vi "medAFMprel.vi"(6 "stop":bool, 8 "error in (no error)":errorcluster, 9 "Tipo":enum16{"Amplitud", "Fase", "Mixto"}(ring), 10 "thrAng":dbl=4.0 format="%#_13g", 11 "thr":dbl) -> (0 "error out":errorcluster, 2 "posicion":dbl)   [LabVIEW 2018]
uses:
  <vilib>/Analysis/NI_AALPro.lvlib
panel:
  out "Cerca":bool
  in  "NUMERO DE MED.":i32=1 min=1 max=10
  in  "wait afm":u32=300
  out "Amplitud":dbl[](graph)=[0.0001737, 0.0001907, 0.0001951, 0.0001957, 0.0001958, 0.0001961, 0.0001961, 0.000196, 0.0001957, 0.0001957, 0.000196, 0.000196, 0.0001958, 0.000196, 0.000196, 0.0001958, 0.0001957, 0.0001957, 0.000196, 0.0001963, 0.0001963, 0.0001966, 0.0001966, 0.0001963, 0.0001965, 0.0001967, 0.0001966, 0.0001966, 0.0001966, 0.0001968, 0.000197, 0.000197, 0.000197, 0.0001968, 0.0001967, 0.0001967, 0.0001966, 0.0001966, 0.0001962, 0.000196, 0.0001961, 0.0001963, 0.0001962, 0.0001962, 0.0001962, 0.0001963, 0.0001965, 0.0001963, 0.0001962, 0.0001961, 0.0001958, 0.0001958, 0.0001958, 0.0001957, 0.0001955, 0.0001955, 0.000196, 0.0001961, 0.0001958, 0.0001956, 0.000196, 0.0001958, 0.0001958, 0.000196, 0.0001958, 0.000196, 0.0001958, 0.0001958, 0.0001958, 0.0001956, 0.0001952, 0.0001952, 0.0001956, 0.0001956, 0.0001957, 0.0001956, 0.0001955, 0.0001958, 0.0001958, 0.0001961, 0.0001962, 0.0001962, 0.0001963, 0.0001966, 0.0001965, 0.0001966, 0.0001966, 0.0001968, 0.0001968, 0.0001966, 0.0001961, 0.0001962, 0.0001965, 0.0001967, 0.0001963, 0.0001961, 0.0001958, 0.0001963, 0.0001966, 0.0001965, 0.0001963, 0.0001961, 0.0001961, 0.0001966, 0.0001968, 0.0001967, 0.0001963, 0.0001961, 0.0001961, 0.0001961, 0.0001958, 0.0001957, 0.0001956, 0.0001957, 0.0001955, 0.0001956, 0.0001958, 0.0001952, 0.0001958, 0.0001958, 0.0001955, 0.0001955, 0.0001955, 0.0001961, 0.0001963, 0.0001965, 0.0001962, 0.000196, 0.0001963, 0.0001966, 0.0001966, 0.0001966, 0.0001963, 0.0001963, 0.0001966, 0.0001966, 0.0001966, 0.0001965, 0.0001963, 0.0001966, 0.0001967, 0.0001968, 0.0001967, 0.0001966, 0.0001966, 0.0001967, 0.0001966, 0.0001965, 0.0001963, 0.0001967, 0.0001963, 0.0001961, 0.0001956, 0.0001956, 0.0001956, 0.0001956, 0.0001955, 0.0001952, 0.0001952, 0.0001952, 0.0001955, 0.0001957, 0.0001956, 0.0001956, 0.0001956, 0.0001957, 0.0001958, 0.0001958, 0.0001956, 0.0001955, 0.0001956, 0.0001958, 0.0001957, 0.0001956, 0.0001956, 0.0001956, 0.0001958, 0.0001957, 0.0001955, 0.0001956, 0.000196, 0.0001958, 0.0001961, 0.000196, 0.000196, 0.0001958, 0.0001965, 0.0001963, 0.0001966, 0.0001965, 0.0001965, 0.0001965, 0.0001963, 0.0001963, 0.0001961, 0.0001961, 0.0001966, 0.0001966, 0.0001966, 0.0001965, 0.0001958, 0.000196, 0.0001962, 0.0001962, 0.0001965, 0.0001962, 0.0001963, 0.0001965, 0.0001963, 0.0001965, 0.0001961, 0.0001961, 0.0001961, 0.0001961, 0.0001962, 0.000196, 0.0001956, 0.0001961, 0.0001961, 0.0001958, 0.0001956, 0.0001953, 0.0001953, 0.0001956, 0.0001956, 0.0001953, 0.0001953, 0.0001955, 0.0001956, 0.0001955, 0.0001953, 0.0001952, 0.0001952, 0.0001957, 0.0001958, 0.0001958, 0.0001958, 0.0001958, 0.0001958, 0.0001958, 0.0001956, 0.0001955, 0.0001957, 0.000196, 0.0001961, 0.0001958, 0.0001957, 0.0001957, 0.0001958, 0.0001961, 0.0001961, 0.0001961, 0.0001958, 0.0001958, 0.0001961, 0.0001965, 0.0001963, 0.0001965, 0.0001965, 0.0001965, 0.0001962, 0.0001963, 0.0001963, 0.0001961, 0.0001961, 0.0001958, 0.0001958, 0.000196, 0.0001958, 0.0001955, 0.0001956, 0.0001958, 0.0001956, 0.0001955, 0.0001957, 0.0001958, 0.0001958, 0.0001958, 0.0001956, 0.0001953, 0.0001953, 0.0001955, 0.0001953, 0.000195, 0.0001947, 0.0001948, 0.0001951, 0.0001951, 0.000195, 0.0001946, 0.0001948, 0.0001948, 0.0001952, 0.000195, 0.000195, 0.0001953, 0.0001956, 0.0001956, 0.0001958, 0.0001958, 0.0001961, 0.0001961, 0.000196, 0.0001958, 0.000196, 0.0001962, 0.0001965, 0.0001961, 0.000196, 0.0001955, 0.0001975, 0.0001981, 0.0001973, 0.0001966, 0.0001957, 0.0001953, 0.0001948, 0.0001946, 0.0001942, 0.0001933, 0.0001905, 0.0001845, 0.0001812, 0.0001717]
  out "Fase":dbl[](graph)=[1.35, -1.7, -2.3, -2.4, -2.4, -2.4, -2.35, -2.4, -2.4, -2.45, -2.45, -2.45, -2.45, -2.4, -2.4, -2.4, -2.4, -2.4, -2.45, -2.4, -2.4, -2.4, -2.4, -2.4, -2.45, -2.45, -2.45, -2.45, -2.5, -2.45, -2.4, -2.45, -2.4, -2.4, -2.4, -2.4, -2.45, -2.4, -2.45, -2.5, -2.5, -2.5, -2.45, -2.45, -2.5, -2.5, -2.45, -2.45, -2.45, -2.45, -2.45, -2.45, -2.45, -2.45, -2.5, -2.5, -2.45, -2.45, -2.45, -2.5, -2.5, -2.45, -2.4, -2.4, -2.4, -2.4, -2.45, -2.45, -2.45, -2.45, -2.5, -2.45, -2.45, -2.45, -2.4, -2.45, -2.5, -2.45, -2.5, -2.5, -2.55, -2.45, -2.45, -2.45, -2.45, -2.45, -2.45, -2.45, -2.45, -2.4, -2.45, -2.45, -2.45, -2.45, -2.45, -2.55, -2.6, -2.5, -2.5, -2.45, -2.5, -2.55, -2.6, -2.55, -2.45, -2.45, -2.45, -2.5, -2.5, -2.55, -2.45, -2.45, -2.45, -2.55, -2.5, -2.45, -2.55, -2.55, -2.5, -2.45, -2.5, -2.5, -2.5, -2.5, -2.45, -2.45, -2.45, -2.55, -2.55, -2.5, -2.5, -2.5, -2.55, -2.55, -2.5, -2.5, -2.5, -2.55, -2.55, -2.55, -2.55, -2.55, -2.55, -2.45, -2.55, -2.5, -2.5, -2.45, -2.5, -2.55, -2.5, -2.5, -2.55, -2.55, -2.55, -2.55, -2.55, -2.6, -2.65, -2.6, -2.55, -2.45, -2.45, -2.5, -2.55, -2.55, -2.55, -2.55, -2.5, -2.6, -2.55, -2.65, -2.55, -2.55, -2.55, -2.5, -2.6, -2.55, -2.55, -2.6, -2.6, -2.6, -2.55, -2.6, -2.6, -2.6, -2.65, -2.6, -2.55, -2.55, -2.55, -2.55, -2.5, -2.55, -2.6, -2.65, -2.7, -2.65, -2.65, -2.65, -2.7, -2.7, -2.6, -2.65, -2.65, -2.65, -2.6, -2.6, -2.55, -2.65, -2.65, -2.6, -2.6, -2.55, -2.55, -2.55, -2.6, -2.6, -2.55, -2.6, -2.6, -2.65, -2.6, -2.65, -2.55, -2.6, -2.55, -2.55, -2.6, -2.6, -2.6, -2.65, -2.6, -2.6, -2.6, -2.6, -2.65, -2.6, -2.6, -2.5, -2.55, -2.6, -2.7, -2.65, -2.6, -2.65, -2.7, -2.7, -2.7, -2.6, -2.55, -2.55, -2.6, -2.65, -2.6, -2.55, -2.6, -2.7, -2.7, -2.65, -2.6, -2.6, -2.6, -2.6, -2.55, -2.6, -2.65, -2.6, -2.65, -2.55, -2.5, -2.5, -2.55, -2.55, -2.6, -2.6, -2.65, -2.65, -2.6, -2.65, -2.65, -2.65, -2.65, -2.7, -2.65, -2.6, -2.6, -2.55, -2.55, -2.55, -2.65, -2.6, -2.65, -2.6, -2.65, -2.65, -2.65, -2.65, -2.65, -2.65, -2.6, -2.6, -2.6, -2.65, -2.65, -2.7, -2.65, -2.6, -2.55, 1.85, 14.25, 17.75, 19.65, 21.45, 22.75, 23.6, 24.45, 25.2, 25.05, 23.35, 15.35, 3.05, 0.4, 7.4]
  out "err R":dbl=0.1226366888094022
  out "diff Ph":dbl=9.8
  out "Z":dbl
  in  "controlP":T1
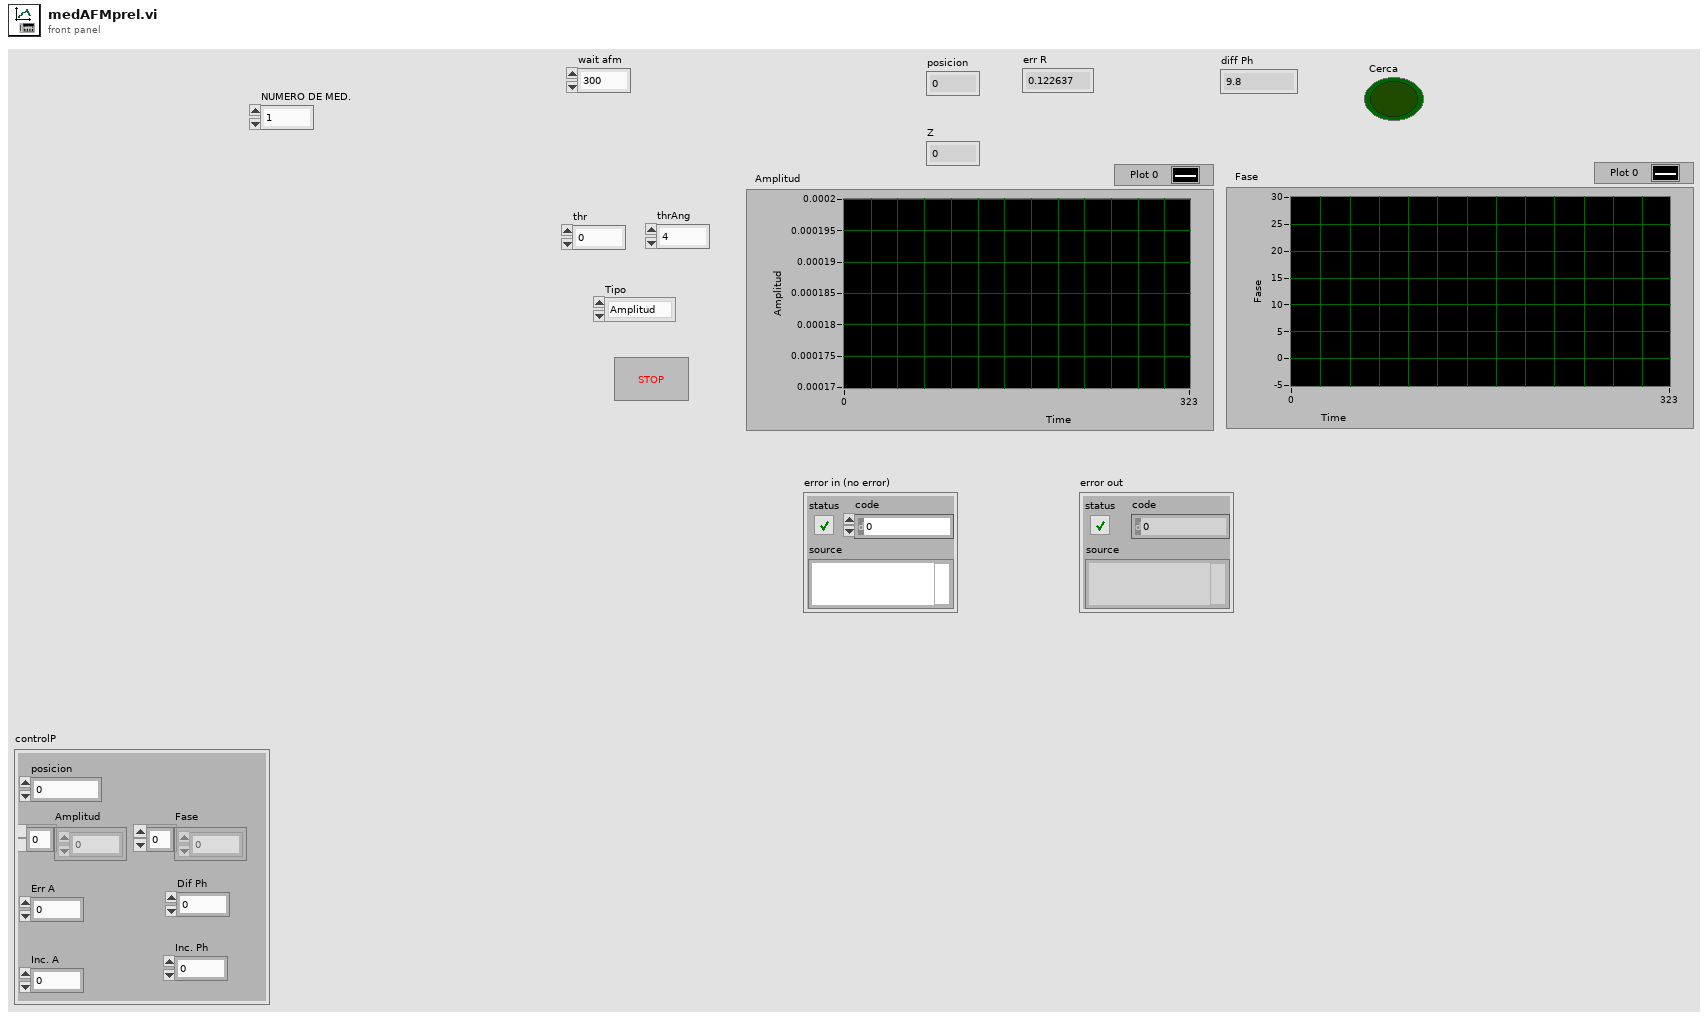
[diagram p1: front panel]
types:
  T1 = cluster{"posicion":dbl, "Amplitud":dbl[], "Fase":dbl[], "Err A":dbl, "Dif Ph":dbl, "Inc. A":dbl, "Inc. Ph":dbl}
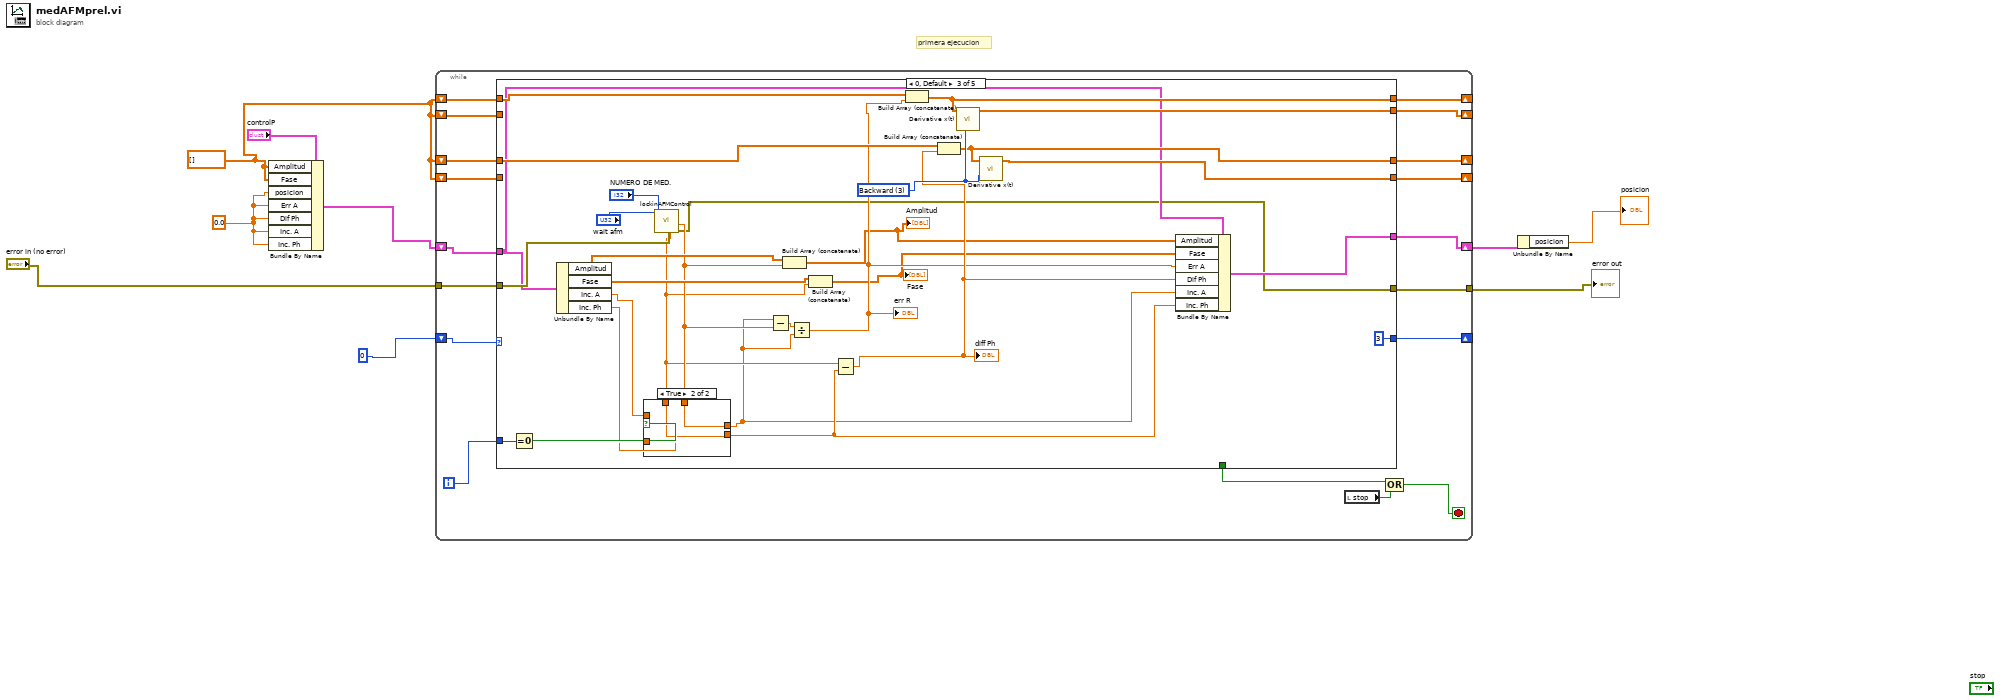
[diagram p0: block diagram]
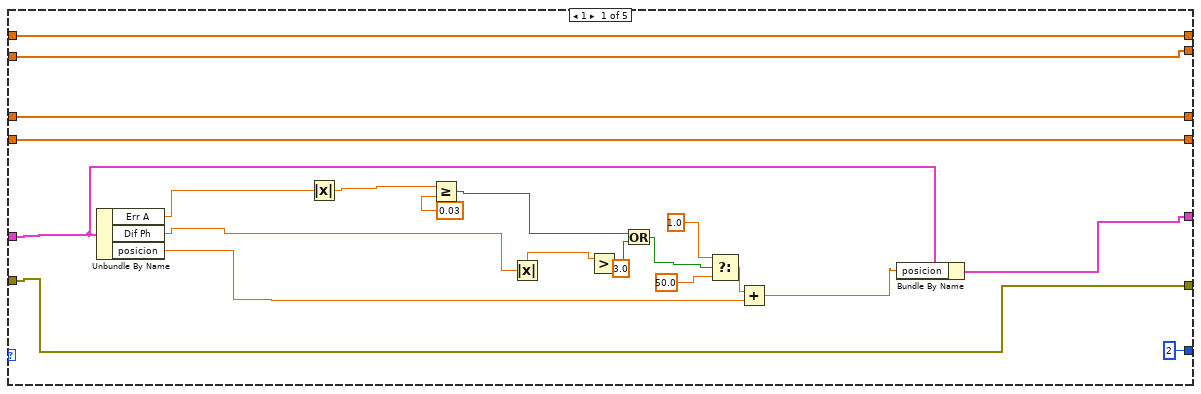
[diagram p2: hidden frame]
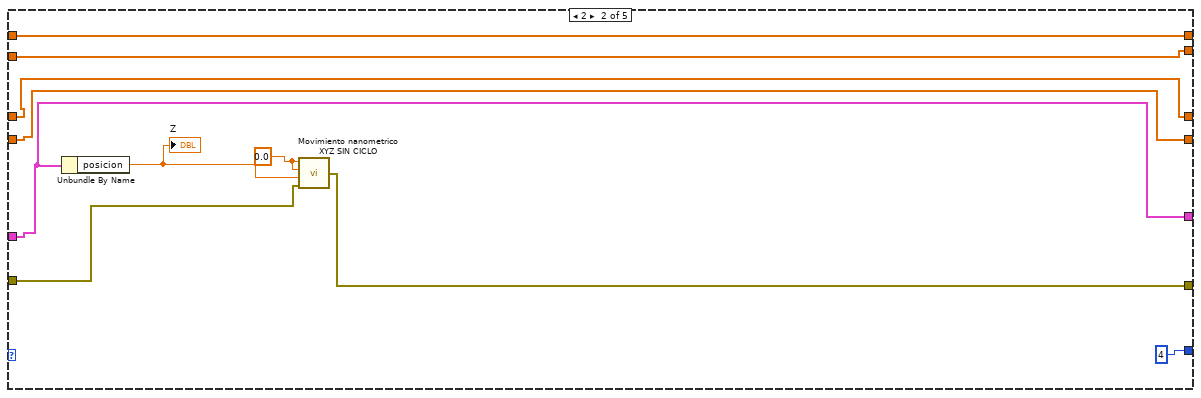
[diagram p3: hidden frame]
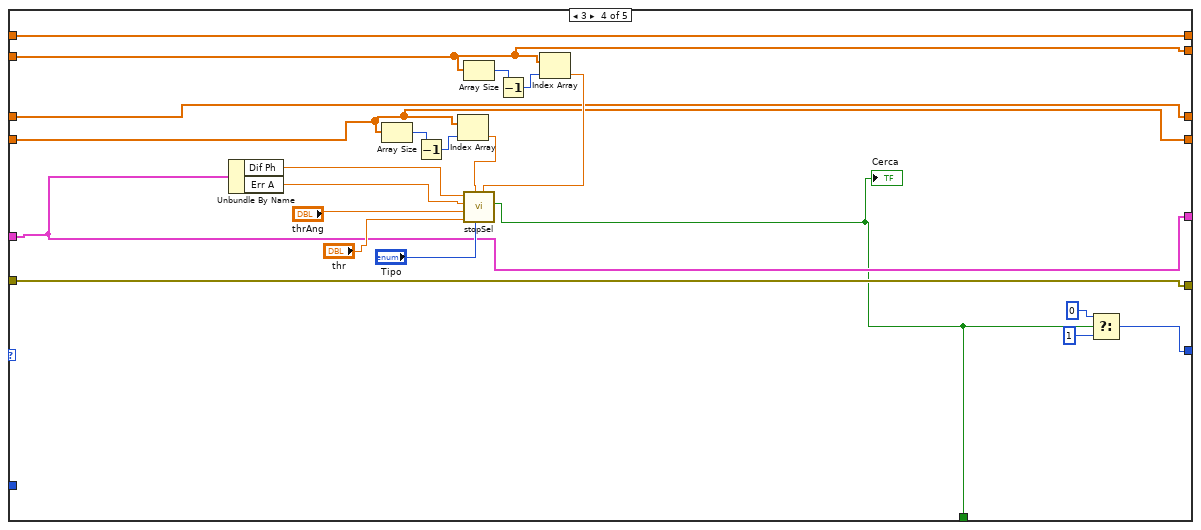
[diagram p5: hidden frame]
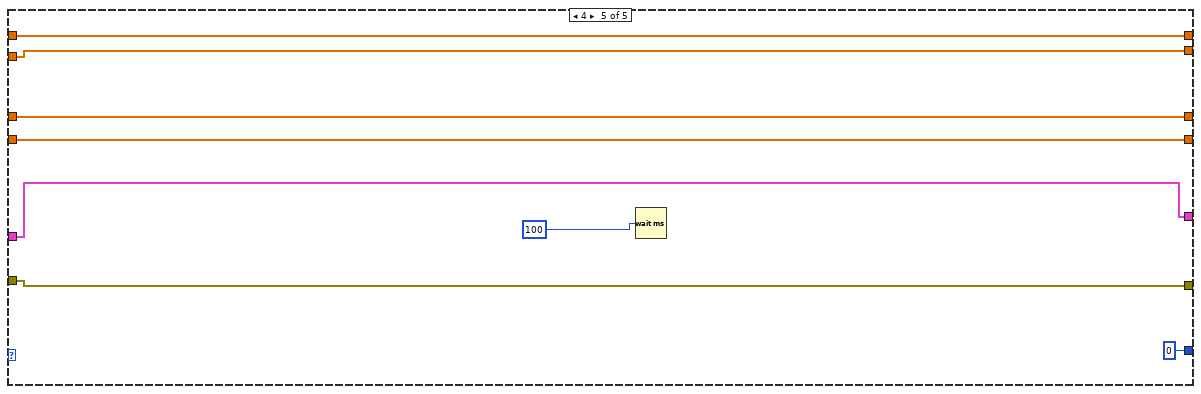
[diagram p6: hidden frame]
diagram:
  w6 = dbl[] []
  w8 = 0.0
  # "primera ejecucion"
  n1 = Bundle By Name(cluster="controlP", "Amplitud"=w6, "Fase"=w6, "posicion"=w8, "Err A"=w8, "Dif Ph"=w8, "Inc. A"=w8, "Inc. Ph"=w8) -> (w7:T1)
  n2 = while {
    shift-right: [w21] -> w4
    shift-left: w7 -> [w26]
    shift-right: [w16] -> _
    shift-left: w6 -> [w22]
    shift-right: [w15] -> _
    shift-left: w6 -> [w23]
    shift-right: [w14] -> _
    shift-left: w6 -> [w24]
    shift-right: [w13] -> _
    shift-left: w6 -> [w25]
    shift-right: [w18] -> _
    shift-left: 0 -> [w27]
    tunnel: "error in (no error)" -> [w20]
    tunnel: [w19] -> w2
    i -> [w17]
    stop <- w10 stop-if-true
    n3 = case shown="0, Default" w27 {
      tunnel: w26 -> [w36 w58 w69 w98 w115]
      tunnel: w25 -> [w29 w51 _ w99 w116]
      tunnel: w24 -> [w30 w52 w72 w100 w117]
      tunnel: w23 -> [w31 w53 _ w101 w118]
      tunnel: w22 -> [w32 w54 w78 w102 w119]
      tunnel: [w34 w58 w62 w98 w115] -> w21
      tunnel: w20 -> [w33 w57 w86 w97 w114]
      tunnel: [w33 w56 w61 w97 w114] -> w19
      tunnel: [2 ("f") 4 3 ("f") w96 0 ("f")] -> w18
      tunnel: w17 -> [_ _ w85 _ _]
      tunnel: [w32 w54 w76 w102 w119] -> w16
      tunnel: [w31 w53 w75 w101 w118] -> w15
      tunnel: [w30 w52 w71 w100 w117] -> w14
      tunnel: [w29 w51 w70 w99 w116] -> w13
      tunnel: [_ _ _ w93 _] -> w11
      frame 1 {
        n4 = Unbundle By Name(w36) -> ("Err A"=w37:dbl, "Dif Ph"=w38:dbl, "posicion"=w39:dbl)
        n5 = Absolute Value(x=w37) -> (abs(x)=w40:dbl)
        n6 = Greater Or Equal?(x=w40, y=0.03) -> (x >= y?=w43:bool)
        n7 = Absolute Value(x=w38) -> (abs(x)=w46:dbl)
        n8 = Greater?(x=w46, y=3.0) -> (0:w42:bool)
        n9 = Or(x=w43, y=w42) -> (x .or. y?=w41:bool)
        n10 = Select(t=1.0, s=w41, f=50.0) -> (s? t:f=w45:dbl)
        n11 = Add(x=w45, y=w39) -> (x+y=w35:dbl)
        n12 = Bundle By Name(cluster=w36, "posicion"=w35) -> (w34:T1)
      }
      frame 2 {
        w59 = 0.0 ("Movimiento en X")
        n13 = Unbundle By Name(w58) -> ("posicion"=w50:dbl)
        "Z" <- w50
        n14 = call "Movimiento nanometrico XYZ SIN CICLO.vi"("Error In"=w57, "Movimiento en Z"=w50, "Movimiento en Y"=w59, "Movimiento en X"=w59) -> ("Error Out"=w56:errorcluster)  [unwired: 2 in]
      }
      frame 0, Default {
        w73 = u16 3 items=["2nd Order Central", "4th Order Central", "Forward", "Backward"] ("method")
        n15 = Equal To 0?(x=w85) -> (x = 0?=w84:bool)
        n16 = Unbundle By Name(w69) -> ("Amplitud"=w81:dbl[], "Fase"=w80:dbl[], "Inc. A"=w82:dbl, "Inc. Ph"=w83:dbl)
        n17 = call "lockinAFMControl.vi"("error in"=w86, "NUMERO DE MED."="NUMERO DE MED.", "milliseconds to wait"="wait afm") -> ("error out"=w61:errorcluster, "Prom. X"=w79:dbl, "Prom. Y"=w74:dbl)  [unwired: 4 in, 2 out]
        n18 = case shown="True" w84 {
          tunnel: w74 -> [_ w91]
          tunnel: [w90 w92] -> w67
          tunnel: w79 -> [_ w92]
          tunnel: [w89 w91] -> w68
          tunnel: w82 -> [w90 _]
          tunnel: w83 -> [w89 _]
          frame False {
          }
          frame True {
          }
        }
        n19 = Subtract(x=w67, y=w79) -> (x-y=w77:dbl)
        n20 = Build Array (concatenate)(w81, w79) -> (w64:dbl[])
        "Amplitud" <- w64
        n21 = Divide(x=w77, y=w67) -> (x/y=w65:dbl)
        "err R" <- w65
        n22 = Build Array (concatenate)(w80, w74) -> (w63:dbl[])
        "Fase" <- w63
        n23 = Subtract(x=w74, y=w68) -> (x-y=w66:dbl)
        "diff Ph" <- w66
        n24 = Build Array (concatenate)(w78, w65) -> (w76:dbl[])
        n25 = Build Array (concatenate)(w72, w66) -> (w71:dbl[])
        n26 = call <vilib>:"Derivative x(t).vi"("method"=w73, "X"=w76) -> ("dX/dt"=w75:dbl[])  [unwired: 8 in, 1 out]
        n27 = call <vilib>:"Derivative x(t).vi"("method"=w73, "X"=w71) -> ("dX/dt"=w70:dbl[])  [unwired: 8 in, 1 out]
        n28 = Bundle By Name(cluster=w69, "Amplitud"=w64, "Fase"=w63, "Err A"=w65, "Dif Ph"=w66, "Inc. A"=w67, "Inc. Ph"=w68) -> (w62:T1)
      }
      frame 3 {
        n29 = Unbundle By Name(w98) -> ("Dif Ph"=w110:dbl, "Err A"=w109:dbl)
        n30 = Array Size(array=w99) -> (size(s)=w108:i32)
        n31 = Decrement(x=w108) -> (x-1=w107:i32)
        n32 = Index Array(array=w99, index=w107) -> (element=w106:dbl)
        n33 = Array Size(array=w101) -> (size(s)=w105:i32)
        n34 = Decrement(x=w105) -> (x-1=w104:i32)
        n35 = Index Array(array=w101, index=w104) -> (element=w103:dbl)
        n36 = call "stopSel.vi"("Der Ampl"=w103, "Tipo"="Tipo", "Der Fase"=w106, "thr"="thr", "thr. Ang"="thrAng", "Err.Amp"=w109, "DifFase"=w110) -> ("stop"=w93:bool)  [unwired: 4 in]
        "Cerca" <- w93
        n37 = Select(t=0, s=w93, f=1) -> (s? t:f=w96:i32)
      }
      frame 4 {
        n38 = Wait (ms)(milliseconds to wait=i64 100) -> ()  [unwired: 1 out]
      }
    }
    n39 = local read "stop"() -> (w12:bool)
    n40 = Compound Arithmetic op=OR(w11, w12) -> (w10:bool)
  }
  "error out" <- w2
  n41 = Unbundle By Name(w4) -> ("posicion"=→"posicion":dbl)
